vi "CSM - No-Event Structure Template.vi"(7 "Name(\"\" to use uuid)":string="JKISM-Module") -> ()   [LabVIEW 2014]
doc: "Template for building CSM Module without User Interface.\n\n<b>Inputs:</b>\n- <b>Name(\"\" to use uuid)</b>: Module Name\n - If Input is \"\", an uuid will be used for module name. The module is marked as stand-alone mode and will not be included in module list.\n - If Input end with '#', the module will worked in worker mode. Modules with the same name will shared the same message queue. Any external message will be processed by one of the modules, depends on who is free.\n - Otherwise, the input string will be used as module name, which should be unique in system. CSM will go to \"Critical Error\" state if duplicated module name is used in system.\n\n<b>Outputs:</b>\n - N/A"
uses:
  _Support/JKISMQ/_Obtain CSMQ.vi
  _Support/FGV-BroadcastRegistry/Cache-Broadcast Registry Search Result.vi
  AdvanceAPI/CSM - Register Status Change.vi
  AdvanceAPI/CSM - Unregister Status Change.vi
  _Support/JKISMQ/_Create Resp Queue.vi
  _Support/JKISMQ/_Unlock CSMQ.vi
  _Support/JKISMQ/_Lock State CSMQ.vi
  _Support/JKISMQ/_Release CSMQ.vi
  AdvanceAPI/CSM - Make String Arguments Safe.vi
  _Support/JKISMQ/_Input Name to CSM Mode.vi
  Utility/uuid.vi
  _Support/KeyWords.vi
  _Support/JKISMQ/_CSMQFGV.vi
  _Support/JKISMQ/_Enqueue CSMQ.vi
  _Support/FGV-BroadcastRegistry/FGV-BroadcastRegistry.vi
  _Support/FGV-BroadcastRegistry/global-Broadcast Cache Change Flag.vi
  _Support/GlobalEvent/FGV-StatusChangeEventRef.vi
  _Support/JKISMQ/_Dequeue CSMQ.vi
  _Support/GlobalEvent/FGV-GlobalEventRef.vi
  Communicable State Machine.lvlib
panel:
  out "Error Occurred":errorcluster
  out "State History":string
  in  "Exit":bool
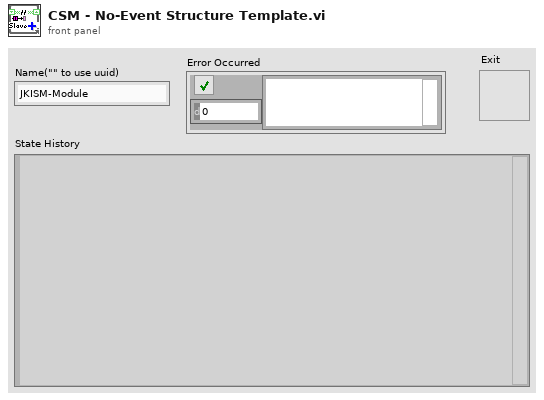
[diagram p1: front panel]
types:
  T1 = enum32{"Invalid", "Standard", "Closed", "Hidden", "Minimized", "Maximized"}
  T2 = enum32{"invalid app kind", "Development System", "Run Time System", "Student Edition", "Embedded LabVIEW", "Evaluation", "Custom"}
  T3 = cluster{"Core":cluster{"Current VI Reference":refnum<vi>, "Close Panel on Exit?":bool}, "Your Boolean data":bool, "Your string data":string}
  T4 = cluster{"Current VI Reference":refnum<vi>, "Close Panel on Exit?":bool}
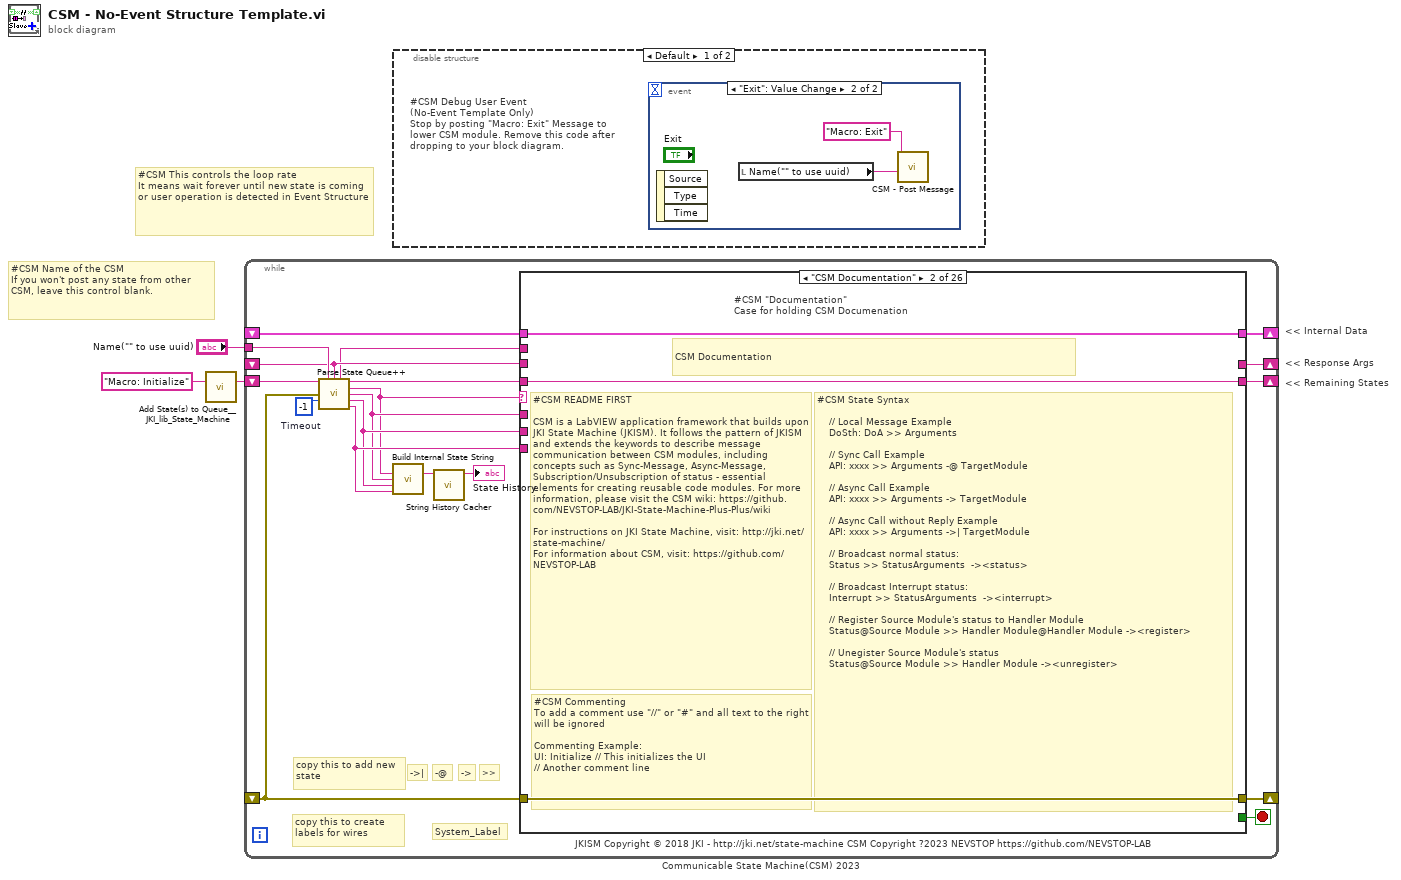
[diagram p0: block diagram]
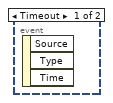
[diagram p2: hidden frame]
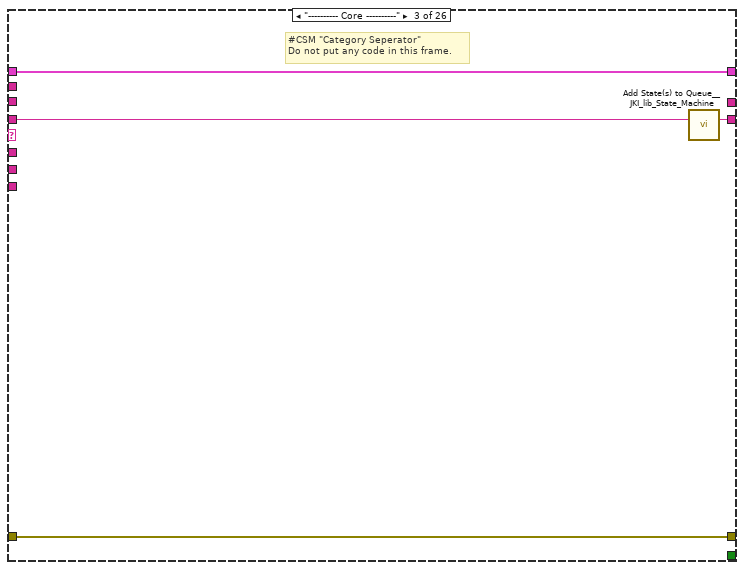
[diagram p5: hidden frame]
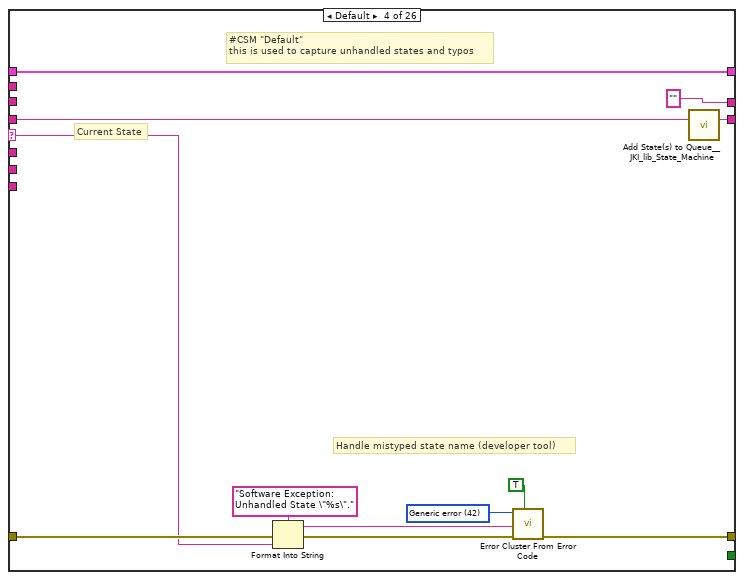
[diagram p6: hidden frame]
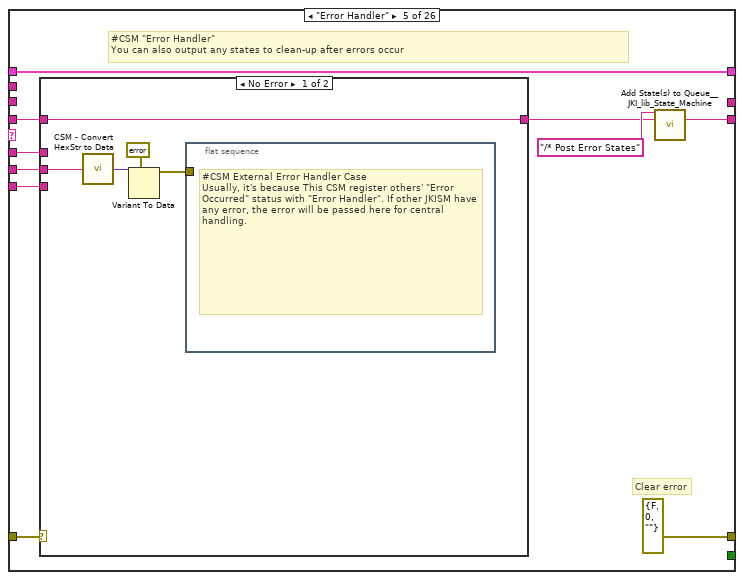
[diagram p7: hidden frame]
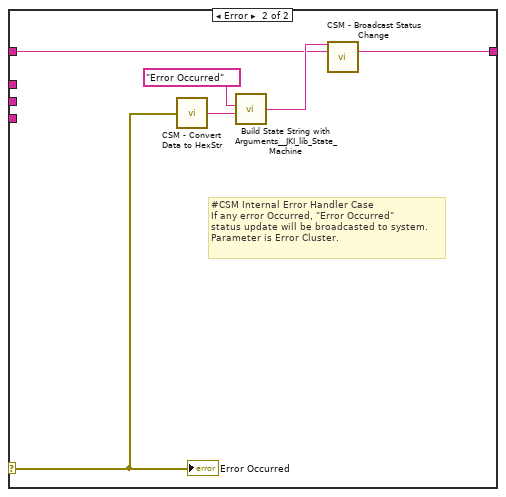
[diagram p8: hidden frame]
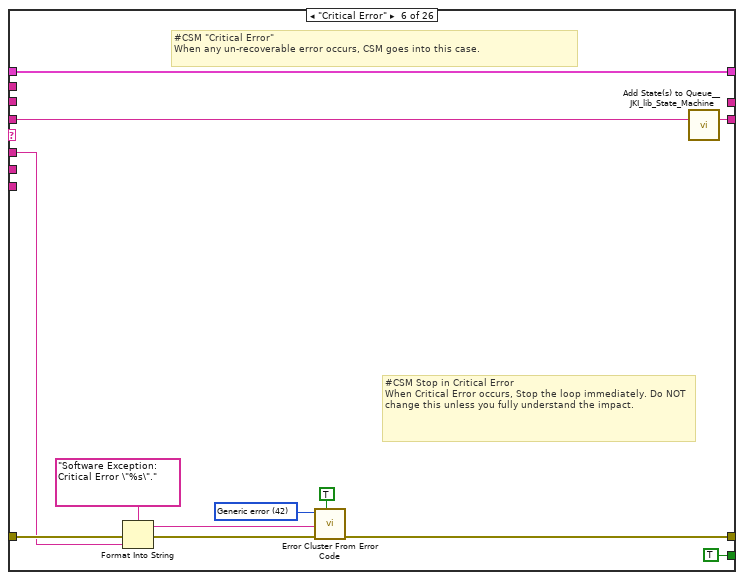
[diagram p9: hidden frame]
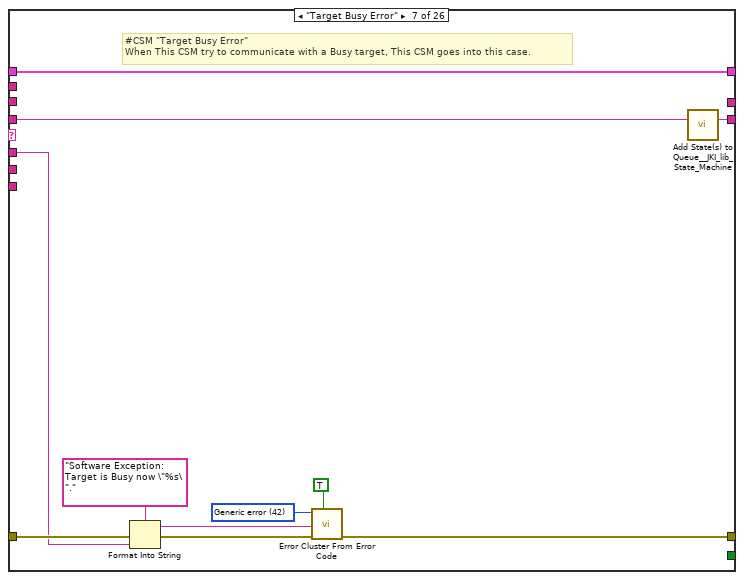
[diagram p10: hidden frame]
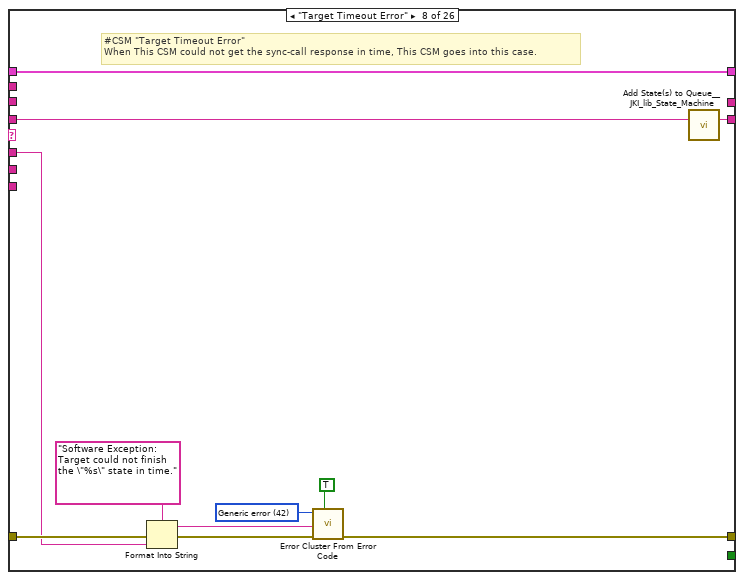
[diagram p11: hidden frame]
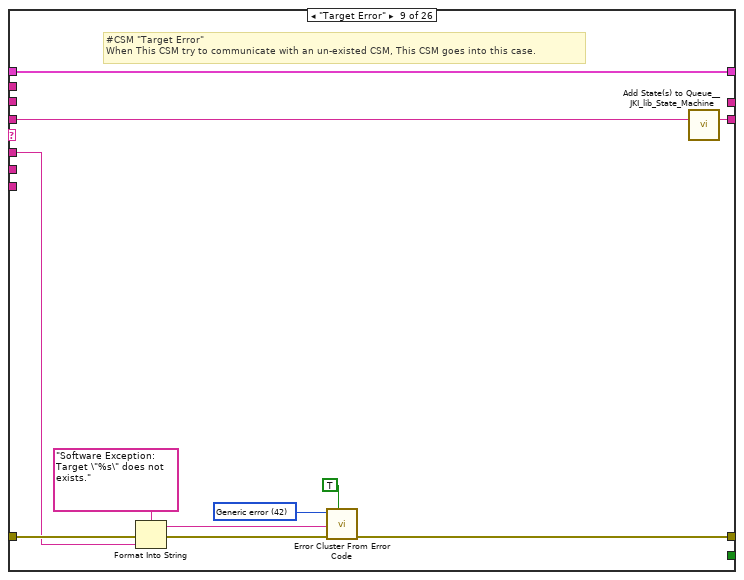
[diagram p12: hidden frame]
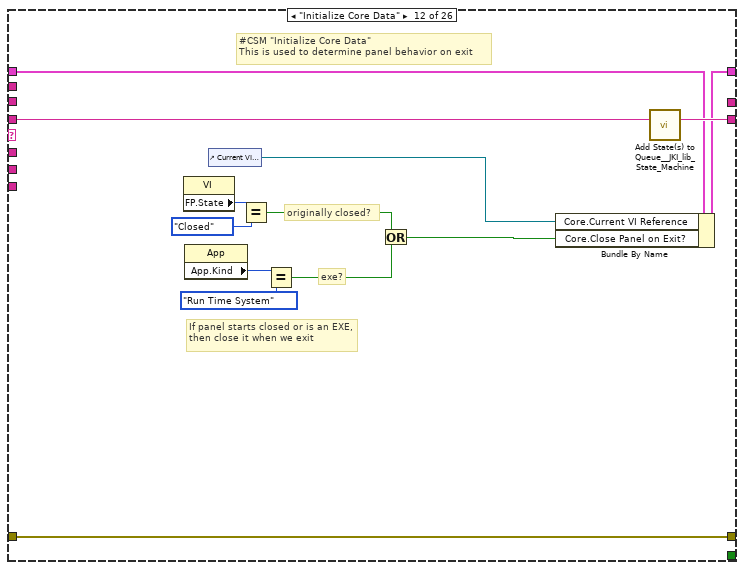
[diagram p15: hidden frame]
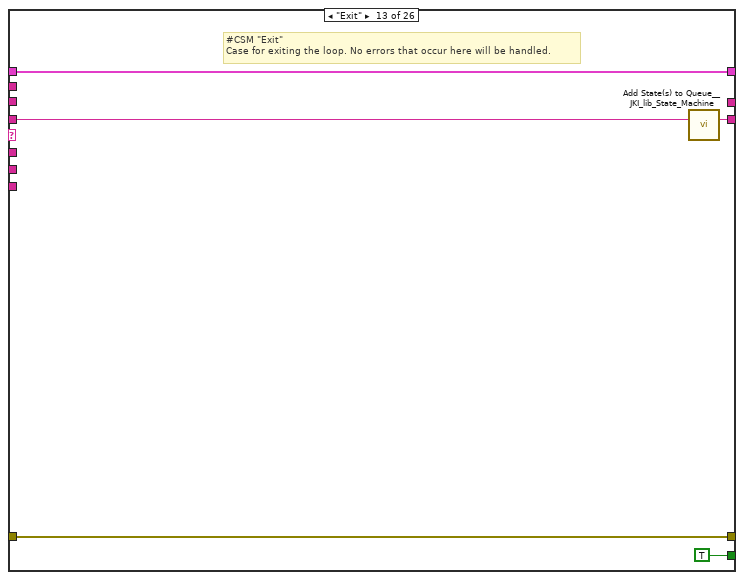
[diagram p16: hidden frame]
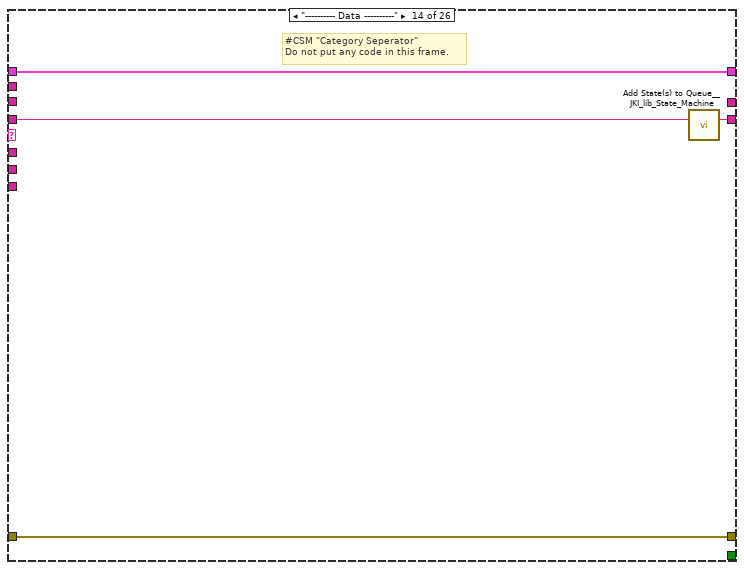
[diagram p17: hidden frame]
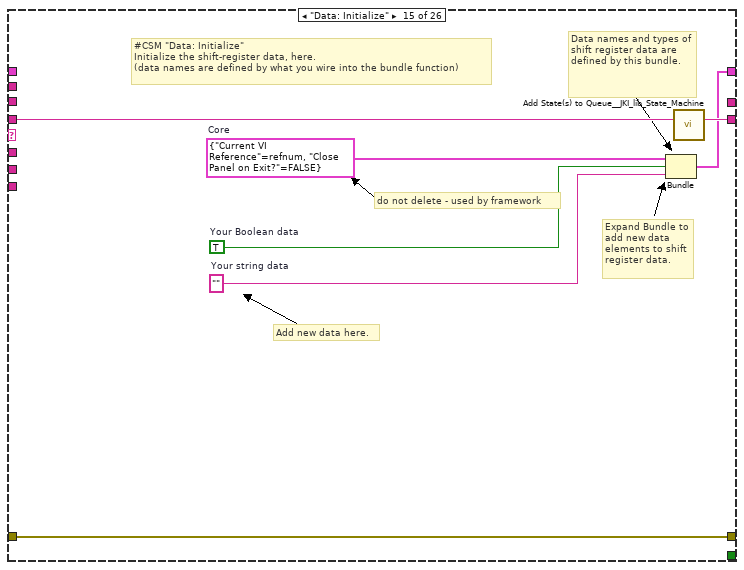
[diagram p18: hidden frame]
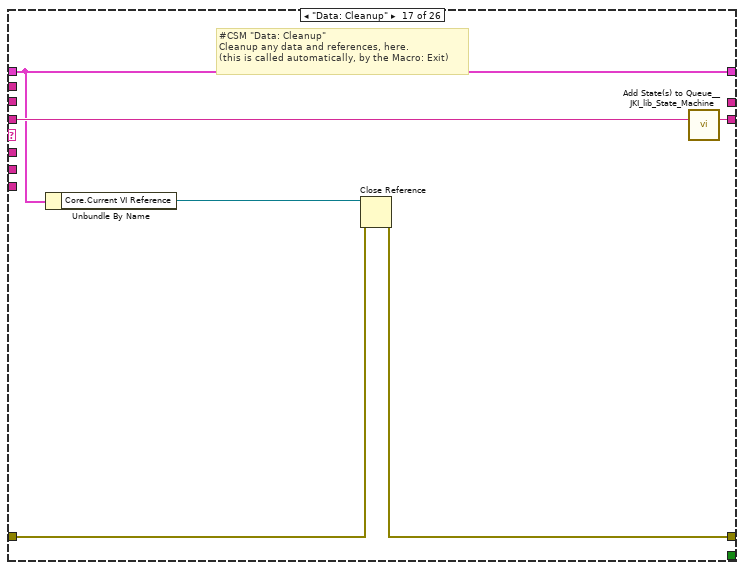
[diagram p20: hidden frame]
diagram:
  # "#CSM Name of the CSM\nIf you won't post any state from other CSM, leave this control blank."
  # "#CSM This controls the loop rate\nIt means wait forever until new state is coming or user operation is detected in Event Structure"
  # "<< Internal Data"
  # "<< Response Args"
  # "<< Remaining States"
  n1 = call <vilib>:"Add State(s) to Queue__JKI_lib_State_Machine.vi"("State(s) in (\"\")"="Macro: Initialize") -> ("States Out"=w3:string)  [unwired: 14 in]
  n2 = while "Communicable State Machine(CSM) 2023" {
    shift-right: [w17] -> _
    shift-left: _ -> [w16]
    shift-right: [w20] -> _
    shift-left: _ -> [w4]
    shift-right: [w19] -> _
    shift-left: w3 -> [w21]
    tunnel: "Name(\"\" to use uuid)" -> [w13]
    shift-right: [w14] -> _
    shift-left: _ -> [w6]
    stop <- w18 stop-if-true
    w15 = -1  # Timeout
    # "->|"
    # "copy this to add new state"
    # ">>"
    # "->"
    # "-@"
    # "JKISM Copyright © 2018 JKI - http://jki.net/state-machine CSM Copyright ?2023 NEVSTOP https://github.com/NEVSTOP-LAB"
    # "copy this to create labels for wires"
    # "System_Label"
    n3 = call "Parse State Queue++.vi"("State Queue"=w21, "Name(\"\" to use uuid)"=w13, "Response Arguments"=w6, "Error In (no error)"=w4, "Dequeue Timeout(0ms)"=w15) -> ("Name Used"=w5:string, "Remaining States"=w22:string, "Current State"=w7:string, "Arguments"=w8:string, "Argument - State"=w9:string, "From Who"=w10:string)  [unwired: 5 in]
    n4 = call "Build Internal State String.vi"("State"=w7, "Arguments (\"\")"=w8, "Arg-State (\"\")"=w9, "Source (\"\")"=w10) -> ("State with Arguments"=w11:string)  [unwired: 11 in]
    n5 = call "String History Cacher.vi"("String"=w11) -> ("String Cache"=→"State History":string)  [unwired: 10 in]
    n6 = case shown="\"CSM Documentation\"" w7 {
      selector: w7 -> [_ _ _ w34 _ _ _ _ _ _ _ _ _ _ _ _ _ _ _ _ _ _ _ _ _ _]
      tunnel: w22 -> [w23 w27 w32 w38 w48 w71 w83 w94 w105 w112 w115 w129 w134 w138 w145 w147 w154 w158 w163 w168 w170 w174 w179 w186 w191 w196]
      tunnel: w8 -> [_ _ _ _ w47 w67 w79 w90 w101 _ _ _ _ _ _ _ _ _ _ _ _ _ w177 _ _ _]
      tunnel: w16 -> [w24 w26 w29 w36 w53 w69 w81 w92 w103 w111 w114 w122 w132 w135 _ w146 w149 w155 w160 w165 w169 w173 w178 w183 w188 w193]
      tunnel: [w25 w28 w30 w40 errorcluster {"status"=FALSE, "code"=0, "source"=""} ("error out") w73 w78 w89 w100 w113 w116 w126 w131 w136 w142 w148 w150 w156 w161 w166 w171 w175 w180 w184 w189 w194] -> w20
      tunnel: w4 -> [w25 w28 w30 w39 w51 w72 w84 w95 w106 w113 w116 w126 w131 w136 w142 w148 w151 w156 w161 w166 w171 w175 w180 w184 w189 w194]
      tunnel: [w23 w27 w31 w37 w49 w70 w82 w93 w104 w112 w115 w128 w133 w137 w144 w147 w153 w157 w162 w167 w170 w174 w179 w185 w190 w195] -> w19
      tunnel: [_ _ _ _ _ TRUE _ _ _ _ _ _ TRUE _ _ _ _ _ _ _ _ _ _ _ _ _] -> w18
      tunnel: [w24 w26 w29 w36 w53 w69 w81 w92 w103 w111 w114 w127 w132 w135 w143 w146 w149 w155 w160 w165 w169 w173 w178 w183 w188 w193] -> w17
      tunnel: w10 -> [_ _ _ _ w46 _ _ _ _ _ _ _ _ _ _ _ _ _ _ _ _ _ _ _ _ _]
      tunnel: w9 -> [_ _ _ _ w45 _ _ _ _ _ _ _ _ _ _ _ _ _ _ _ _ _ _ _ _ _]
      tunnel: [_ _ _ "" _ _ _ _ _ _ _ _ _ _ _ _ _ _ _ _ _ "API1 Response" w176 _ "DoA Finished" "DoB Finished"] -> w14
      tunnel: w5 -> [_ _ _ _ _ _ _ _ _ _ _ _ _ _ _ _ _ _ _ _ _ _ _ _ _ _]
      tunnel: w6 -> [_ _ _ _ _ _ _ _ _ _ _ _ _ _ _ _ _ _ _ _ _ _ _ _ _ _]
      frame "", "Idle" {
        # "#CSM \"Idle/Event Handler\"\nexecutes when the state queue is empty"
      }
      frame "CSM Documentation" {
        # "CSM Documentation"
        # "#CSM Commenting\nTo add a comment use \"//\" or \"#\" and all text to the right will be ignored\n\nCommenting Example:\nUI: Initialize // This initializes the UI\n// Another comment line"
        # "#CSM State Syntax\n\n    // Local Message Example\n    DoSth: DoA >> Arguments\n\n    // Sync Call Example\n    API: xxxx >> Arguments -@ TargetModule\n\n    // Async Call Example\n    API: xxxx >> Arguments -> TargetModule\n\n    // Async Call without Reply Example\n    API: xxxx >> Arguments ->| TargetModule\n\n    // Broadcast normal status:\n    Status >> StatusArguments  -><status>\n\n    // Broadcast Interrupt status:\n    Interrupt >> StatusArguments  -><interrupt>\n\n    // Register Source Module's status to Handler Module\n    Status@Source Module >> Handler Module@Handler Module -><register>\n\n    // Unegister Source Module's status\n    Status@Source Module >> Handler Module -><unregister>"
        # "#CSM README FIRST\n\nCSM is a LabVIEW application framework that builds upon JKI State Machine (JKISM). It follows the pattern of JKISM and extends the keywords to describe message communication between CSM modules, including concepts such as Sync-Message, Async-Message, Subscription/Unsubscription of status - essential elements for creating reusable code modules. For more information, please visit the CSM wiki: https://github.com/NEVSTOP-LAB/JKI-State-Machine-Plus-Plus/wiki\n\nFor instructions on JKI State Machine, visit: http://jki.net/state-machine/\nFor information about CSM, visit: https://github.com/NEVSTOP-LAB"
        # "#CSM \"Documentation\"\nCase for holding CSM Documenation"
      }
      frame "---------- Core ----------" {
        # "#CSM \"Category Seperator\"\nDo not put any code in this frame."
        n7 = call <vilib>:"Add State(s) to Queue__JKI_lib_State_Machine.vi"("State(s) in (\"\")"=w32) -> ("States Out"=w31:string)  [unwired: 14 in]
      }
      frame Default {
        w43 = 42 items=["No error", "Argument error", "Memory is full", "Out of zone", "End of file", "File already open", "Generic file I/O error", "File not found", "File permission error", "Disk is full", "Duplicate path", "Too many files open", "System feature not enabled", "Resource file not found", "Cannot add resource", "Resource not found", "Image not found", "Image memory error", "Pen does not exist", "Config type invalid", "Config token not found", "Config parse error", "Config memory error", "Bad external code format", "Bad external code offset", "External code not present", "Null window", "Destroy window error", "Null menu", "Print aborted", "Bad print record", "Print driver error", "Windows error during printing", "Memory error during printing", "Print dialog error", "Generic print error", "Invalid device refnum", "Device not found", "Device parameter error", "Device unit error", "Cannot open device", "Device call aborted", "Generic error", "Cancelled by user", "Object ID too low", "Object ID too high", "Object not in heap", "Unknown heap", "Unknown object (invalid DefProc)", "Unknown object (DefProc not in table)", "Message out of range", "Invalid (null) method", "Unknown message", "Manager call not supported", "Bad address", "Network operation in progress", "Network operation timed out", "Connection is busy", "Network attribute not supported", "Network error", "Address in use", "System out of memory", "Connection aborted", "Connection refused", "Not connected", "Already connected", "Connection closed", "Initialization error (interapplication manager)", "Bad occurrence", "Wait on unbound occurrence handler", "Occurrence queue overflow", "Datalog type conflict", "Unused", "Unrecognized type (interapplication manager)", "Memory corrupt", "Failed to make temporary DLL", "Old CIN version", "Drag socket not found", "Failed to load drop-object", "Failed to register OLE object", "Failed to release OLE object", "Format specifier type mismatch", "Unknown format specifier", "Too few format specifiers", "Too many format specifiers", "Scan failed", "Newer CIN version", "Error converting to variant", "Runtime menu error", "Password tampered", "Variant attribute not found", "Incompatible variant data type", "Event data is not available", "Event Store is not present", "Occurrence is not found", "Event Queue is not created", "Event info is not available", "Refnum passed is NULL", "Error retrieving Class GUID", "Error retrieving CoClass GUID", "Error retrieving TypeLib GUID.", "Bad built application magic bytes.", "Specific driver is different from the specific driver associated with the Logical Name.", "There is no session opened to the class driver.", "Max Error", "MAX - Error with config objects", "MAX - Error loading configuration", "MAX - Group not supported"]
        # "#CSM \"Default\"\nthis is used to capture unhandled states and typos"
        # "Current State"
        # "Handle mistyped state name (developer tool)"
        n8 = Format Into String(format string="Software Exception: Unhandled State \"%s\"." ("message"), error in=w39, w34) -> (resulting string=w42:string, error out=w41:errorcluster)  [unwired: 1 in]
        n9 = call <vilib>:"Error Cluster From Error Code.vi"("show call chain? (False)"=TRUE, "error in (no error)"=w41, "error message (\"\")"=w42, "error code (0)"=w43) -> ("error out"=w40:errorcluster)  [unwired: 5 in]
        n10 = call <vilib>:"Add State(s) to Queue__JKI_lib_State_Machine.vi"("State(s) in (\"\")"=w38) -> ("States Out"=w37:string)  [unwired: 14 in]
      }
      frame "Error Handler" {
        # "#CSM \"Error Handler\"\nYou can also output any states to clean-up after errors occur"
        # "Clear error"
        n11 = case shown="No Error" w51 {
          selector: w51 -> [_ w63]
          tunnel: [w59 w61] -> w50
          tunnel: w48 -> [w59 w60]
          tunnel: w47 -> [_ _]
          tunnel: w46 -> [_ _]
          tunnel: w45 -> [w58 _]
          frame No Error {
            n12 = call "CSM - Convert HexStr to Data.vi"("HEX String"=w58) -> ("Variant"=w57:variant)  [unwired: 7 in, 1 out]
            n13 = Variant To Data(type=errorcluster {"status"=FALSE, "code"=0, "source"=""} ("error in (no error)"), Variant=w57) -> (data=w55:errorcluster)  [unwired: 1 in, 1 out]
            n14 = flat-sequence {
              tunnel: w55 -> [_]
              frame #0 {
                # "#CSM External Error Handler Case\nUsually, it's because This CSM register others' \"Error Occurred\" status with \"Error Handler\". If other JKISM have any error, the error will be passed here for central handling."
              }
            }
          }
          frame Error {
            # "#CSM Internal Error Handler Case \nIf any error Occurred, \"Error Occurred\" \nstatus update will be broadcasted to system.\nParameter is Error Cluster."
            n15 = call "CSM - Convert Data to HexStr.vi"("Variant"=w63) -> ("HEX String (0-9,A-F)"=w64:string)  [unwired: 8 in]
            n16 = call <vilib>:"Build State String with Arguments__JKI_lib_State_Machine.vi"("Arguments (\"\")"=w64, "State"="Error Occurred" ("Status with Arguments")) -> ("State with Arguments"=w62:string)  [unwired: 4 in]
            n17 = call "CSM - Broadcast Status Change.vi"("Status with Arguments"=w62, "State Queue"=w60) -> ("Remaining States"=w61:string)  [unwired: 13 in]
            "Error Occurred" <- w63
          }
        }
        n18 = call <vilib>:"Add State(s) to Queue__JKI_lib_State_Machine.vi"("State(s) in Front (\"\")"="/* Post Error States", "State(s) in (\"\")"=w50) -> ("States Out"=w49:string)  [unwired: 13 in]
      }
      frame "Critical Error" {
        w76 = 42 items=["No error", "Argument error", "Memory is full", "Out of zone", "End of file", "File already open", "Generic file I/O error", "File not found", "File permission error", "Disk is full", "Duplicate path", "Too many files open", "System feature not enabled", "Resource file not found", "Cannot add resource", "Resource not found", "Image not found", "Image memory error", "Pen does not exist", "Config type invalid", "Config token not found", "Config parse error", "Config memory error", "Bad external code format", "Bad external code offset", "External code not present", "Null window", "Destroy window error", "Null menu", "Print aborted", "Bad print record", "Print driver error", "Windows error during printing", "Memory error during printing", "Print dialog error", "Generic print error", "Invalid device refnum", "Device not found", "Device parameter error", "Device unit error", "Cannot open device", "Device call aborted", "Generic error", "Cancelled by user", "Object ID too low", "Object ID too high", "Object not in heap", "Unknown heap", "Unknown object (invalid DefProc)", "Unknown object (DefProc not in table)", "Message out of range", "Invalid (null) method", "Unknown message", "Manager call not supported", "Bad address", "Network operation in progress", "Network operation timed out", "Connection is busy", "Network attribute not supported", "Network error", "Address in use", "System out of memory", "Connection aborted", "Connection refused", "Not connected", "Already connected", "Connection closed", "Initialization error (interapplication manager)", "Bad occurrence", "Wait on unbound occurrence handler", "Occurrence queue overflow", "Datalog type conflict", "Unused", "Unrecognized type (interapplication manager)", "Memory corrupt", "Failed to make temporary DLL", "Old CIN version", "Drag socket not found", "Failed to load drop-object", "Failed to register OLE object", "Failed to release OLE object", "Format specifier type mismatch", "Unknown format specifier", "Too few format specifiers", "Too many format specifiers", "Scan failed", "Newer CIN version", "Error converting to variant", "Runtime menu error", "Password tampered", "Variant attribute not found", "Incompatible variant data type", "Event data is not available", "Event Store is not present", "Occurrence is not found", "Event Queue is not created", "Event info is not available", "Refnum passed is NULL", "Error retrieving Class GUID", "Error retrieving CoClass GUID", "Error retrieving TypeLib GUID.", "Bad built application magic bytes.", "Specific driver is different from the specific driver associated with the Logical Name.", "There is no session opened to the class driver.", "Max Error", "MAX - Error with config objects", "MAX - Error loading configuration", "MAX - Group not supported"]
        # "#CSM \"Critical Error\"\nWhen any un-recoverable error occurs, CSM goes into this case."
        # "#CSM Stop in Critical Error\nWhen Critical Error occurs, Stop the loop immediately. Do NOT change this unless you fully understand the impact."
        n19 = Format Into String(format string="Software Exception: Critical Error \"%s\"." ("message"), error in=w72, w67) -> (resulting string=w75:string, error out=w74:errorcluster)  [unwired: 1 in]
        n20 = call <vilib>:"Error Cluster From Error Code.vi"("show call chain? (False)"=TRUE, "error in (no error)"=w74, "error message (\"\")"=w75, "error code (0)"=w76) -> ("error out"=w73:errorcluster)  [unwired: 5 in]
        n21 = call <vilib>:"Add State(s) to Queue__JKI_lib_State_Machine.vi"("State(s) in (\"\")"=w71) -> ("States Out"=w70:string)  [unwired: 14 in]
      }
      frame "Target Busy Error" {
        w87 = 42 items=["No error", "Argument error", "Memory is full", "Out of zone", "End of file", "File already open", "Generic file I/O error", "File not found", "File permission error", "Disk is full", "Duplicate path", "Too many files open", "System feature not enabled", "Resource file not found", "Cannot add resource", "Resource not found", "Image not found", "Image memory error", "Pen does not exist", "Config type invalid", "Config token not found", "Config parse error", "Config memory error", "Bad external code format", "Bad external code offset", "External code not present", "Null window", "Destroy window error", "Null menu", "Print aborted", "Bad print record", "Print driver error", "Windows error during printing", "Memory error during printing", "Print dialog error", "Generic print error", "Invalid device refnum", "Device not found", "Device parameter error", "Device unit error", "Cannot open device", "Device call aborted", "Generic error", "Cancelled by user", "Object ID too low", "Object ID too high", "Object not in heap", "Unknown heap", "Unknown object (invalid DefProc)", "Unknown object (DefProc not in table)", "Message out of range", "Invalid (null) method", "Unknown message", "Manager call not supported", "Bad address", "Network operation in progress", "Network operation timed out", "Connection is busy", "Network attribute not supported", "Network error", "Address in use", "System out of memory", "Connection aborted", "Connection refused", "Not connected", "Already connected", "Connection closed", "Initialization error (interapplication manager)", "Bad occurrence", "Wait on unbound occurrence handler", "Occurrence queue overflow", "Datalog type conflict", "Unused", "Unrecognized type (interapplication manager)", "Memory corrupt", "Failed to make temporary DLL", "Old CIN version", "Drag socket not found", "Failed to load drop-object", "Failed to register OLE object", "Failed to release OLE object", "Format specifier type mismatch", "Unknown format specifier", "Too few format specifiers", "Too many format specifiers", "Scan failed", "Newer CIN version", "Error converting to variant", "Runtime menu error", "Password tampered", "Variant attribute not found", "Incompatible variant data type", "Event data is not available", "Event Store is not present", "Occurrence is not found", "Event Queue is not created", "Event info is not available", "Refnum passed is NULL", "Error retrieving Class GUID", "Error retrieving CoClass GUID", "Error retrieving TypeLib GUID.", "Bad built application magic bytes.", "Specific driver is different from the specific driver associated with the Logical Name.", "There is no session opened to the class driver.", "Max Error", "MAX - Error with config objects", "MAX - Error loading configuration", "MAX - Group not supported"]
        # "#CSM \"Target Busy Error\"\nWhen This CSM try to communicate with a Busy target, This CSM goes into this case."
        n22 = Format Into String(format string="Software Exception: Target is Busy now \"%s\"." ("message"), error in=w84, w79) -> (resulting string=w86:string, error out=w85:errorcluster)  [unwired: 1 in]
        n23 = call <vilib>:"Error Cluster From Error Code.vi"("show call chain? (False)"=TRUE, "error in (no error)"=w85, "error message (\"\")"=w86, "error code (0)"=w87) -> ("error out"=w78:errorcluster)  [unwired: 5 in]
        n24 = call <vilib>:"Add State(s) to Queue__JKI_lib_State_Machine.vi"("State(s) in (\"\")"=w83) -> ("States Out"=w82:string)  [unwired: 14 in]
      }
      frame "Target Timeout Error" {
        w98 = 42 items=["No error", "Argument error", "Memory is full", "Out of zone", "End of file", "File already open", "Generic file I/O error", "File not found", "File permission error", "Disk is full", "Duplicate path", "Too many files open", "System feature not enabled", "Resource file not found", "Cannot add resource", "Resource not found", "Image not found", "Image memory error", "Pen does not exist", "Config type invalid", "Config token not found", "Config parse error", "Config memory error", "Bad external code format", "Bad external code offset", "External code not present", "Null window", "Destroy window error", "Null menu", "Print aborted", "Bad print record", "Print driver error", "Windows error during printing", "Memory error during printing", "Print dialog error", "Generic print error", "Invalid device refnum", "Device not found", "Device parameter error", "Device unit error", "Cannot open device", "Device call aborted", "Generic error", "Cancelled by user", "Object ID too low", "Object ID too high", "Object not in heap", "Unknown heap", "Unknown object (invalid DefProc)", "Unknown object (DefProc not in table)", "Message out of range", "Invalid (null) method", "Unknown message", "Manager call not supported", "Bad address", "Network operation in progress", "Network operation timed out", "Connection is busy", "Network attribute not supported", "Network error", "Address in use", "System out of memory", "Connection aborted", "Connection refused", "Not connected", "Already connected", "Connection closed", "Initialization error (interapplication manager)", "Bad occurrence", "Wait on unbound occurrence handler", "Occurrence queue overflow", "Datalog type conflict", "Unused", "Unrecognized type (interapplication manager)", "Memory corrupt", "Failed to make temporary DLL", "Old CIN version", "Drag socket not found", "Failed to load drop-object", "Failed to register OLE object", "Failed to release OLE object", "Format specifier type mismatch", "Unknown format specifier", "Too few format specifiers", "Too many format specifiers", "Scan failed", "Newer CIN version", "Error converting to variant", "Runtime menu error", "Password tampered", "Variant attribute not found", "Incompatible variant data type", "Event data is not available", "Event Store is not present", "Occurrence is not found", "Event Queue is not created", "Event info is not available", "Refnum passed is NULL", "Error retrieving Class GUID", "Error retrieving CoClass GUID", "Error retrieving TypeLib GUID.", "Bad built application magic bytes.", "Specific driver is different from the specific driver associated with the Logical Name.", "There is no session opened to the class driver.", "Max Error", "MAX - Error with config objects", "MAX - Error loading configuration", "MAX - Group not supported"]
        # "#CSM \"Target Timeout Error\"\nWhen This CSM could not get the sync-call response in time, This CSM goes into this case."
        n25 = Format Into String(format string="Software Exception: Target could not finish the \"%s\" state in time." ("message"), error in=w95, w90) -> (resulting string=w97:string, error out=w96:errorcluster)  [unwired: 1 in]
        n26 = call <vilib>:"Error Cluster From Error Code.vi"("show call chain? (False)"=TRUE, "error in (no error)"=w96, "error message (\"\")"=w97, "error code (0)"=w98) -> ("error out"=w89:errorcluster)  [unwired: 5 in]
        n27 = call <vilib>:"Add State(s) to Queue__JKI_lib_State_Machine.vi"("State(s) in (\"\")"=w94) -> ("States Out"=w93:string)  [unwired: 14 in]
      }
      frame "Target Error" {
        w109 = 42 items=["No error", "Argument error", "Memory is full", "Out of zone", "End of file", "File already open", "Generic file I/O error", "File not found", "File permission error", "Disk is full", "Duplicate path", "Too many files open", "System feature not enabled", "Resource file not found", "Cannot add resource", "Resource not found", "Image not found", "Image memory error", "Pen does not exist", "Config type invalid", "Config token not found", "Config parse error", "Config memory error", "Bad external code format", "Bad external code offset", "External code not present", "Null window", "Destroy window error", "Null menu", "Print aborted", "Bad print record", "Print driver error", "Windows error during printing", "Memory error during printing", "Print dialog error", "Generic print error", "Invalid device refnum", "Device not found", "Device parameter error", "Device unit error", "Cannot open device", "Device call aborted", "Generic error", "Cancelled by user", "Object ID too low", "Object ID too high", "Object not in heap", "Unknown heap", "Unknown object (invalid DefProc)", "Unknown object (DefProc not in table)", "Message out of range", "Invalid (null) method", "Unknown message", "Manager call not supported", "Bad address", "Network operation in progress", "Network operation timed out", "Connection is busy", "Network attribute not supported", "Network error", "Address in use", "System out of memory", "Connection aborted", "Connection refused", "Not connected", "Already connected", "Connection closed", "Initialization error (interapplication manager)", "Bad occurrence", "Wait on unbound occurrence handler", "Occurrence queue overflow", "Datalog type conflict", "Unused", "Unrecognized type (interapplication manager)", "Memory corrupt", "Failed to make temporary DLL", "Old CIN version", "Drag socket not found", "Failed to load drop-object", "Failed to register OLE object", "Failed to release OLE object", "Format specifier type mismatch", "Unknown format specifier", "Too few format specifiers", "Too many format specifiers", "Scan failed", "Newer CIN version", "Error converting to variant", "Runtime menu error", "Password tampered", "Variant attribute not found", "Incompatible variant data type", "Event data is not available", "Event Store is not present", "Occurrence is not found", "Event Queue is not created", "Event info is not available", "Refnum passed is NULL", "Error retrieving Class GUID", "Error retrieving CoClass GUID", "Error retrieving TypeLib GUID.", "Bad built application magic bytes.", "Specific driver is different from the specific driver associated with the Logical Name.", "There is no session opened to the class driver.", "Max Error", "MAX - Error with config objects", "MAX - Error loading configuration", "MAX - Group not supported"]
        # "#CSM \"Target Error\"\nWhen This CSM try to communicate with an un-existed CSM, This CSM goes into this case."
        n28 = Format Into String(format string="Software Exception: Target \"%s\" does not exists." ("message"), error in=w106, w101) -> (resulting string=w108:string, error out=w107:errorcluster)  [unwired: 1 in]
        n29 = call <vilib>:"Error Cluster From Error Code.vi"("show call chain? (False)"=TRUE, "error in (no error)"=w107, "error message (\"\")"=w108, "error code (0)"=w109) -> ("error out"=w100:errorcluster)  [unwired: 5 in]
        n30 = call <vilib>:"Add State(s) to Queue__JKI_lib_State_Machine.vi"("State(s) in (\"\")"=w105) -> ("States Out"=w104:string)  [unwired: 14 in]
      }
      frame "Async Response", "Response" {
        # "#CSM Response Comments\nAfter Message is executed, CSM goes to this state for receive the response.\n    For Async Message(->), \"Async Response\" is used. This CSM will goes to \"Async Message Posted\" immediately and receive the \"Async Response\" after the callee finishes the message.\n    For Sync Message(@),  This CSM will wait until the message is done and immediately goes to \"Response\""
        # "#CSM \"Async Response\"\nHandle Async-call Response (\"Async Response\" for ->)"
        # "#CSM \"Response\"\nHandle Sync-call Response (\"Response\" for -@)"
      }
      frame "Async Message Posted" {
        # "#CSM \"Async Message Posted\"\nAfter Async Message is posted (-> or ->| ), CSM goes to this state for post-action.\nYou can use Argument - State to tell which Async Message is called."
      }
      frame "Initialize Core Data" {
        # "#CSM \"Initialize Core Data\"\nThis is used to determine panel behavior on exit"
        # "originally closed?"
        # "exe?"
        # "If panel starts closed or is an EXE, then close it when we exit"
        n31 = property class="VI"() -> ("FP.State"=w119:T1)  [unwired: 2 in, 2 out]
        n32 = property class="App"() -> ("App.Kind"=w125:T2)  [unwired: 2 in, 2 out]
        n33 = control-ref of="Current VI Reference"() -> (w120:refnum<vi>)
        n34 = Equal?(x=w119, y=T1."Closed" ("Front Panel Window:State")) -> (x = y?=w117:bool)
        n35 = Equal?(x=w125, y=T2."Run Time System" ("Application:Kind")) -> (x = y?=w123:bool)
        n36 = Or(x=w117, y=w123) -> (x .or. y?=w121:bool)
        n37 = Bundle By Name(cluster=w122, "Core.Current VI Reference"=w120, "Core.Close Panel on Exit?"=w121) -> (w127:T3)
        n38 = call <vilib>:"Add State(s) to Queue__JKI_lib_State_Machine.vi"("State(s) in (\"\")"=w129) -> ("States Out"=w128:string)  [unwired: 14 in]
      }
      frame "Exit" {
        # "#CSM \"Exit\"\nCase for exiting the loop. No errors that occur here will be handled."
        n39 = call <vilib>:"Add State(s) to Queue__JKI_lib_State_Machine.vi"("State(s) in (\"\")"=w134) -> ("States Out"=w133:string)  [unwired: 14 in]
      }
      frame "---------- Data ----------" {
        # "#CSM \"Category Seperator\"\nDo not put any code in this frame."
        n40 = call <vilib>:"Add State(s) to Queue__JKI_lib_State_Machine.vi"("State(s) in (\"\")"=w138) -> ("States Out"=w137:string)  [unwired: 14 in]
      }
      frame "Data: Initialize" {
        w139 = T4 {"Current VI Reference"=refnum, "Close Panel on Exit?"=FALSE}  # Core
        w141 = TRUE  # Your Boolean data
        w140 = ""  # Your string data
        # "#CSM \"Data: Initialize\"\nInitialize the shift-register data, here.\n(data names are defined by what you wire into the bundle function)"
        # "do not delete - used by framework"
        # "Expand Bundle to add new data elements to shift register data."
        # "Add new data here."
        # "Data names and types of shift register data are defined by this bundle."
        n41 = Bundle("Core"=w139, "Your Boolean data"=w141, "Your string data"=w140) -> (w143:T3)  [unwired: 1 in]
        n42 = call <vilib>:"Add State(s) to Queue__JKI_lib_State_Machine.vi"("State(s) in (\"\")"=w145) -> ("States Out"=w144:string)  [unwired: 14 in]
      }
      frame "Data: Update Indicators" {
      }
      frame "Data: Cleanup" {
        # "#CSM \"Data: Cleanup\"\nCleanup any data and references, here.\n(this is called automatically, by the Macro: Exit)"
        n43 = Unbundle By Name(w149) -> ("Core.Current VI Reference"=w152:refnum<vi>)
        n44 = Close Reference(reference=w152, error in (no error)=w151) -> (error out=w150:errorcluster)
        n45 = call <vilib>:"Add State(s) to Queue__JKI_lib_State_Machine.vi"("State(s) in (\"\")"=w154) -> ("States Out"=w153:string)  [unwired: 14 in]
      }
      frame "---------- Macro ----------" {
        # "#CSM \"Category Seperator\"\nDo not put any code in this frame."
        n46 = call <vilib>:"Add State(s) to Queue__JKI_lib_State_Machine.vi"("State(s) in (\"\")"=w158) -> ("States Out"=w157:string)  [unwired: 14 in]
      }
      frame "Macro: Initialize" {
        # "#CSM \"Macro: Initialize\"\nInitialization Macro (This is called once, when the VI starts)"
        n47 = call <vilib>:"Add State(s) to Queue__JKI_lib_State_Machine.vi"("State(s) in Front (\"\")"="Data: Initialize\nInitialize Core Data\nData: Update Indicators", "State(s) in (\"\")"=w163) -> ("States Out"=w162:string)  [unwired: 13 in]
      }
      frame "Macro: Exit" {
        # "#CSM \"Macro: Exit\"\nExit Macro (This is called once, when the VI exits)"
        n48 = call <vilib>:"Add State(s) to Queue__JKI_lib_State_Machine.vi"("State(s) in Front (\"\")"="Data: Cleanup\nExit", "State(s) in (\"\")"=w168) -> ("States Out"=w167:string)  [unwired: 13 in]
      }
      frame "---------- API ----------" {
        # "#CSM \"Category Seperator\"\nDo not put any code in this frame."
      }
      frame "API: API1" {
        # "#CSM API Example\nCopy/Rename this case for your own API"
        # "#CSM >> From Who >>\nIf you need to tell who triggered this state , use this string. If it's this case itself, this string is \"\"."
        # "#CSM >> Arguments >>\nDeal with the parameter if any"
        # "#CSM Response\nConnect this to return the response of your API"
      }
      frame "API: API2" {
        # "#CSM API Example\nCopy/Rename this case for your own API"
        # "unpack Hex String  to Variant\nif complex parameter is needed."
        n49 = call "CSM - Convert HexStr to Data.vi"("HEX String"=w177) -> ()  [unwired: 7 in, 2 out]
        n50 = disable-structure shown="Enabled" {
          disable-tunnel: [w181 "API2 Response"] -> w176
          frame Disabled {
            # "pack variant to hexstr \nif complex response is needed."
            # "complex Response"
            n51 = call "CSM - Convert Data to HexStr.vi"() -> ("HEX String (0-9,A-F)"=w181:string)  [unwired: 9 in]
          }
          frame Enabled {
          }
        }
      }
      frame "---------- DoSth ----------" {
        # "#CSM \"Category Seperator\"\nDo not put any code in this frame."
        n52 = call <vilib>:"Add State(s) to Queue__JKI_lib_State_Machine.vi"("State(s) in (\"\")"=w186) -> ("States Out"=w185:string)  [unwired: 14 in]
      }
      frame "DoSth: DoA" {
        # "#CSM \"Internal State\"\nThis category is used for holding internal states"
        n53 = call <vilib>:"Add State(s) to Queue__JKI_lib_State_Machine.vi"("State(s) in (\"\")"=w191) -> ("States Out"=w190:string)  [unwired: 14 in]
      }
      frame "DoSth: DoB" {
        # "#CSM \"Internal State\"\nThis category is used for holding internal states"
        n54 = call <vilib>:"Add State(s) to Queue__JKI_lib_State_Machine.vi"("State(s) in (\"\")"=w196) -> ("States Out"=w195:string)  [unwired: 14 in]
      }
    }
  }
  n55 = disable-structure shown="Default" {
    frame condition #0 (active) {
      # "#CSM Debug User Event\n(No-Event Template Only)\nStop by posting \"Macro: Exit\" Message to lower CSM module. Remove this code after dropping to your block diagram."
      n56 = event shown="[1] \"Exit\": Value Change" {
        selector: _ -> [_ _]
        dyn-events: _ -> [_ _]
        timeout: _ -> [_ _]
        event Timeout {
          n57 = event-data() -> ()  [unwired: 1 in, 3 out]
        }
        event "Exit": Value Change {
          n58 = event-data() -> ()  [unwired: 1 in, 3 out]
          n59 = local read "Name(\"\" to use uuid)"() -> (w198:string)
          n60 = call "CSM - Post Message.vi"("Target Module"=w198, "State"="Macro: Exit" ("States")) -> ()  [unwired: 9 in, 1 out]
        }
      }
    }
    frame condition #1 {
    }
  }
